vi "Measurement UI.vi"() -> ()   [LabVIEW 2024, in "Frequency Response (Discrete Sweep) UI.lvlib"]
uses:
  Frequency Response (Discrete Sweep) UI.lvlib
  <vilib>/gRPC/Generated APIs/ni/protobuf/types/RPC Messages/ni_protobuf_types_DoubleXYData.ctl
  <vilib>/gRPC/Generated APIs/ni/protobuf/types/ni.protobuf.types.lvlib
panel:
  out "RMS levels":cluster{"X":dbl[], "Y":dbl[]}[](graph)
  out "response RMS level":T1
  out "reference RMS level":T1
  out "Magnitude":cluster{"frequency":dbl[], "magnitude":dbl[]}(graph)
  out "FRF magnitude":T1
  out "Phase":cluster{"frequency":dbl[], "magnitude":dbl[]}(graph)
  out "FRF phase":T1
  out "Harmonic Distortion":cluster{"X":dbl[], "Y":dbl[]}[](graph)
  out "THDN":T1
  out "h5":T1
  out "h4":T1
  out "h3":T1
  out "h2":T1
  out "THD":T1
  out "waveforms file path":path
  in  "ai response":T2={"ai response channel (I/O)"="", "range"=3.16, "terminal configuration"=-1} {"terminal configuration" items=["Default"=-1, "RSE"=10083, "NRSE"=10078, "Differential"=10106, "Pseudodifferential"=12529]; "range" format="± %#_6f V"}
  in  "ai reference":T3={"ai reference channel (I/O)"="", "range"=3.16, "terminal configuration"=-1} {"terminal configuration" items=["Default"=-1, "RSE"=10083, "NRSE"=10078, "Differential"=10106, "Pseudodifferential"=12529]; "range" format="± %#_6f V"}
  in  "ao stimulus":T4={"ao stimulus channel (I/O)"="", "range"=3.16, "terminal configuration"=-1} {"terminal configuration" items=["Default"=-1, "RSE"=10083, "Differential"=10106, "Pseudodifferential"=12529]; "range" format="± %#_4f V"}
  in  "ai response terminal configuration":i32(ring)=-1 items=["Default"=-1, "RSE"=10083, "NRSE"=10078, "Differential"=10106, "Pseudodifferential"=12529]
  in  "ai response range":dbl=3.16 format="± %#_6f V"
  in  "ai response channel":string="Dev1/ai1"
  in  "ai reference terminal configuration":i32(ring)=-1 items=["Default"=-1, "RSE"=10083, "NRSE"=10078, "Differential"=10106, "Pseudodifferential"=12529]
  in  "ai ref range":dbl=3.16 format="± %#_6f V"
  in  "ai reference channel":string="Dev1/ai0"
  in  "ao terminal configuration":i32(ring)=-1 items=["Default"=-1, "RSE"=10083, "Differential"=10106, "Pseudodifferential"=12529]
  in  "ao range":dbl=3.16 format="± %#_4f V"
  in  "ao stimulus channel":string="Dev1/ao0"
  in  "sample rate":dbl=51200.0 format="%#_4p Hz"
  in  "amplitude":dbl=1.4142 format="%#_6f V"
  in  "profile":enum32{"Linear", "Logarithmic"}(ring)=enum."Logarithmic"
  in  "number of steps":i32=100 min=1
  in  "stop frequency":dbl=16000.0 format="%.2f Hz"
  in  "start frequency":dbl=31.25 format="%.2f Hz"
  in  "measurement cycles":i32=20 caption="cycles" min=1
  in  "measurement time":dbl=0.01 caption="time" format="%#_4f s"
  out "current frequency":dbl format="%#_g Hz"
  # "DAQ"
  # "Source"
  # "Measurement"
  # "Status"
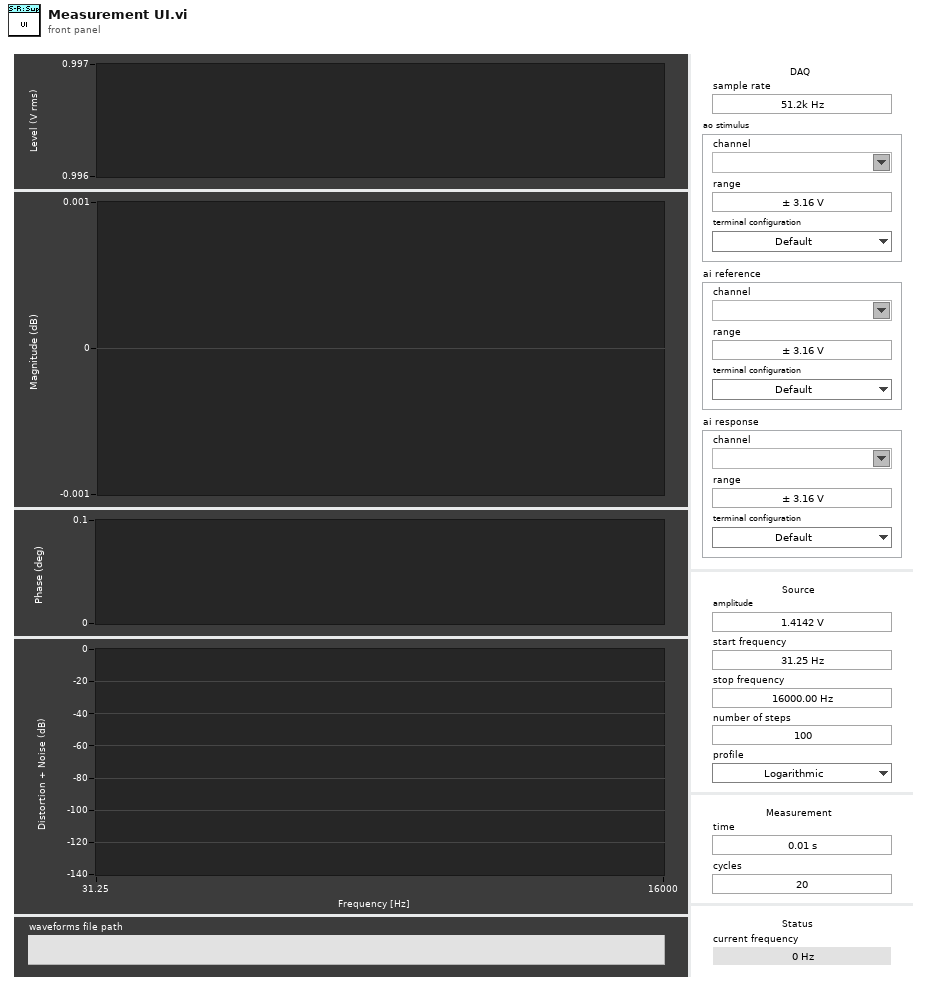
[diagram p1: front panel]
types:
  T1 = typedef "ni.protobuf.types.lvlib/ni_protobuf_types_DoubleXYData.ctl" = cluster{"x_data":dbl[], "y_data":dbl[]}
  T2 = cluster{"ai response channel (I/O)":tag, "range":dbl, "terminal configuration":i32}
  T3 = cluster{"ai reference channel (I/O)":tag, "range":dbl, "terminal configuration":i32}
  T4 = cluster{"ao stimulus channel (I/O)":tag, "range":dbl, "terminal configuration":i32}
  T5 = enum8{"Enabled", "Disabled", "Disabled and Grayed Out"}
  T6 = cluster{"I/O channel":tag, "range":dbl, "terminal configuration":i32}
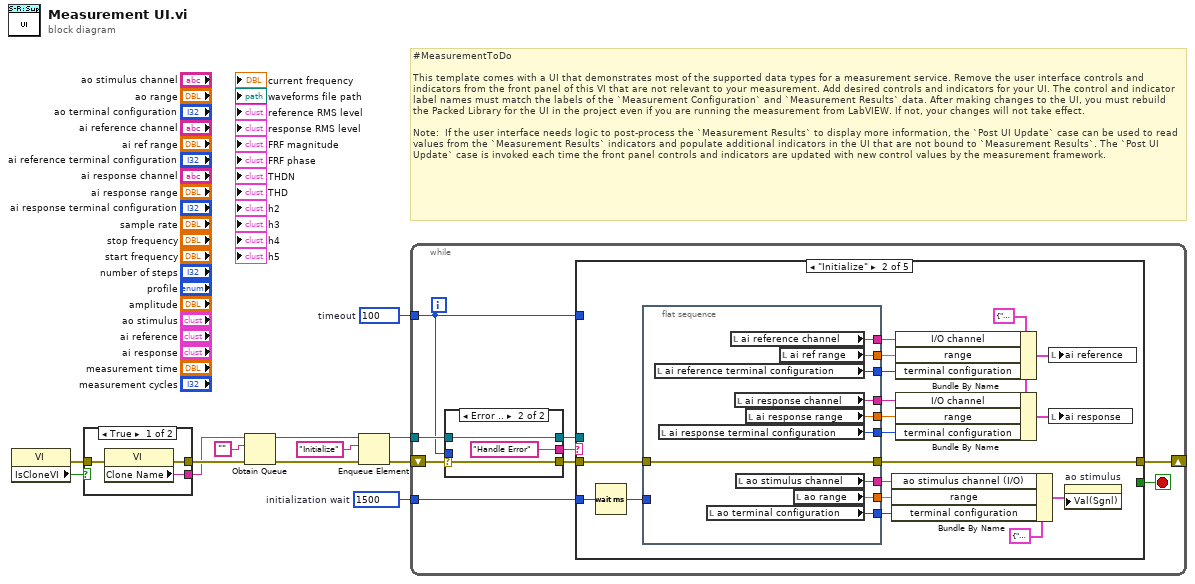
[diagram p0: block diagram]
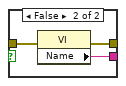
[diagram p2: hidden frame]
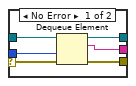
[diagram p3: hidden frame]
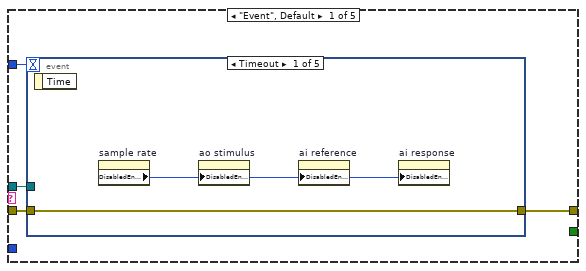
[diagram p4: hidden frame]
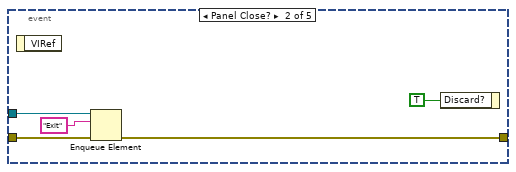
[diagram p5: hidden frame]
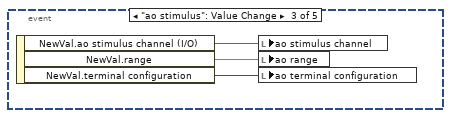
[diagram p6: hidden frame]
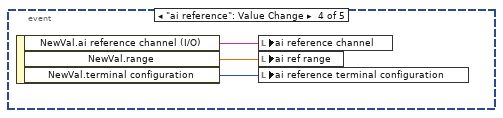
[diagram p7: hidden frame]
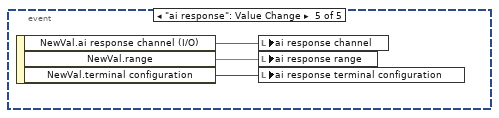
[diagram p8: hidden frame]
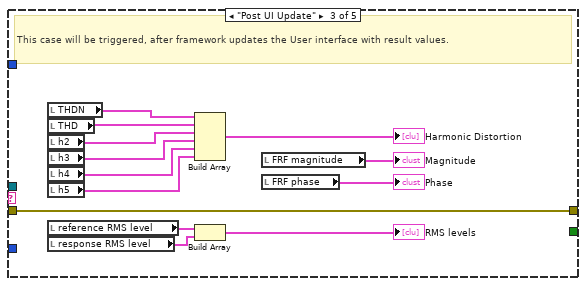
[diagram p9: hidden frame]
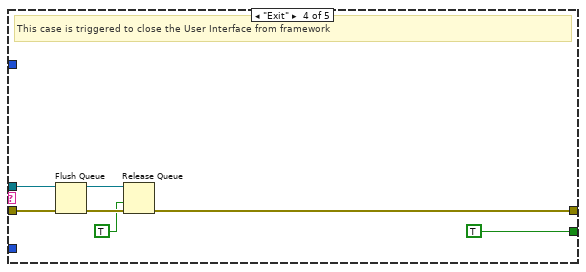
[diagram p10: hidden frame]
diagram:
  w1 = u32 1500  # initialization wait
  w2 = 100  # timeout
  # "#MeasurementToDo  \n\nThis template comes with a UI that demonstrates most of the supported data types for a measurement service. Remove the user interface controls and indicators from the front panel of this VI that are not relevant to your measurement. Add desired controls and indicators for your UI. The control and indicator label names must match the labels of the `Measurement Configuration` and `Measurement Results` data. After making changes to the UI, you must rebuild the Packed Library for the UI in the project even if you are running the measurement from LabVIEW. If not, your changes will not take effect.\n\nNote:  If the user interface needs logic to post-process the `Measurement Results` to display more information, the `Post UI Update` case can be used to read values from the `Measurement Results` indicators and populate additional indicators in the UI that are not bound to `Measurement Results`. The `Post UI Update` case is invoked each time the front panel controls and indicators are updated with new control values by the measurement framework."
  n1 = property class="VI"() -> (error out=w3:errorcluster, "IsCloneVI"=w4:bool)  [unwired: 2 in, 1 out]
  n2 = case shown="True" w4 {
    tunnel: [w15 w18] -> w12
    tunnel: [w14 w17] -> w11
    tunnel: w3 -> [w13 w16]
    frame True {
      n3 = property class="VI"(error in=w13) -> (error out=w15:errorcluster, "Clone Name"=w14:string)  [unwired: 1 in, 1 out]
    }
    frame False {
      n4 = property class="VI"(error in=w16) -> (error out=w18:errorcluster, "Name"=w17:string)  [unwired: 1 in, 1 out]
    }
  }
  n5 = Obtain Queue(name (unnamed)=w11, element data type="", error in (no error)=w12) -> (queue out=w8:refnum<queue>, error out=w10:errorcluster)  [unwired: 2 in, 1 out]
  n6 = Enqueue Element(queue=w8, element="Initialize", error in (no error)=w10) -> (queue out=w7:refnum<queue>, error out=w9:errorcluster)  [unwired: 1 in, 1 out]
  n7 = while {
    shift-right: [w22] -> _
    shift-left: w9 -> [w27]
    tunnel: w7 -> [w25]
    tunnel: w2 -> [w20]
    tunnel: w1 -> [w19]
    stop <- w21 stop-if-true
    n8 = case shown="Error .." w27 {
      selector: w27 -> [w33 w36]
      tunnel: [w32 w36] -> w26
      tunnel: w25 -> [w31 w35]
      tunnel: [w30 w35] -> w24
      tunnel: [w29 "Handle Error"] -> w23
      tunnel: w20 -> [w28 _]
      frame No Error {
        n9 = Dequeue Element(queue=w31, timeout in ms (-1)=w28, error in (no error)=w33) -> (queue out=w30:refnum<queue>, element=w29:string, error out=w32:errorcluster)  [unwired: 1 out]
      }
      frame Error {
      }
    }
    n10 = case shown="\"Initialize\"" w23 {
      tunnel: w26 -> [w39 w59 w97 w104 w105]
      tunnel: w24 -> [w38 _ _ w102 _]
      tunnel: [w40 w60 w97 w99 w105] -> w22
      tunnel: [_ _ _ TRUE _] -> w21
      tunnel: w20 -> [w37 _ _ _ _]
      tunnel: w19 -> [_ w58 _ _ _]
      frame "Event", Default {
        n11 = event shown="[0] Timeout" {
          selector: _ -> [_ _ _ _ _]
          dyn-events: _ -> [_ _ _ _ _]
          timeout: w37 -> [_ _ _ _ _]
          tunnel: [w42 w45 _ _ _] -> w40
          tunnel: w39 -> [w42 w46 _ _ _]
          tunnel: w38 -> [_ w44 _ _ _]
          event Timeout {
            n12 = event-data() -> ()  [unwired: 1 in, 1 out]
            n13 = property on="sample rate" class="DigNum (strict)"() -> ("DisabledEnum"=w41:T5)  [unwired: 2 in, 2 out]
            n14 = property on="ao stimulus" class="Clust (strict)"("DisabledEnum"=w41) -> ()  [unwired: 2 in, 2 out]
            n15 = property on="ai reference" class="Clust (strict)"("DisabledEnum"=w41) -> ()  [unwired: 2 in, 2 out]
            n16 = property on="ai response" class="Clust (strict)"("DisabledEnum"=w41) -> ()  [unwired: 2 in, 2 out]
          }
          event Panel Close? {
            n17 = event-data() -> ()  [unwired: 1 in, 1 out]
            n18 = Enqueue Element(queue=w44, element="Exit", error in (no error)=w46) -> (error out=w45:errorcluster)  [unwired: 1 in, 2 out]
            n19 = event-data("Discard?"=TRUE) -> ()  [unwired: 1 in, 1 out]
          }
          event "ao stimulus": Value Change {
            n20 = event-data() -> ("NewVal.ao stimulus channel (I/O)"=w50:tag, "NewVal.range"=w49:dbl, "NewVal.terminal configuration"=w48:i32)  [unwired: 1 in]
            n21 = local write "ao stimulus channel"(w50) -> ()
            n22 = local write "ao range"(w49) -> ()
            n23 = local write "ao terminal configuration"(w48) -> ()
          }
          event "ai reference": Value Change {
            n24 = event-data() -> ("NewVal.ai reference channel (I/O)"=w53:tag, "NewVal.range"=w52:dbl, "NewVal.terminal configuration"=w51:i32)  [unwired: 1 in]
            n25 = local write "ai reference channel"(w53) -> ()
            n26 = local write "ai ref range"(w52) -> ()
            n27 = local write "ai reference terminal configuration"(w51) -> ()
          }
          event "ai response": Value Change {
            n28 = event-data() -> ("NewVal.ai response channel (I/O)"=w56:tag, "NewVal.range"=w55:dbl, "NewVal.terminal configuration"=w54:i32)  [unwired: 1 in]
            n29 = local write "ai response channel"(w56) -> ()
            n30 = local write "ai response range"(w55) -> ()
            n31 = local write "ai response terminal configuration"(w54) -> ()
          }
        }
      }
      frame "Initialize" {
        w61 = T6 {"I/O channel"="", "range"=31.25, "terminal configuration"=-1} ("ai reference")
        n32 = Wait (ms)(milliseconds to wait=w58) -> (millisecond timer value=w57:u32)
        n33 = flat-sequence {
          tunnel: [w84] -> w73
          tunnel: [w83] -> w72
          tunnel: [w82] -> w71
          tunnel: [w81] -> w69
          tunnel: [w80] -> w67
          tunnel: [w79] -> w66
          tunnel: [w78] -> w65
          tunnel: [w77] -> w64
          tunnel: [w76] -> w62
          tunnel: [w75] -> w60
          tunnel: w59 -> [w75]
          tunnel: w57 -> [_]
          frame #0 {
            n34 = local read "ai reference terminal configuration"() -> (w79:i32)
            n35 = local read "ai response terminal configuration"() -> (w78:i32)
            n36 = local read "ao terminal configuration"() -> (w82:i32)
            n37 = local read "ai reference channel"() -> (w80:string)
            n38 = local read "ai response channel"() -> (w77:string)
            n39 = local read "ao stimulus channel"() -> (w84:string)
            n40 = local read "ai response range"() -> (w76:dbl)
            n41 = local read "ai ref range"() -> (w81:dbl)
            n42 = local read "ao range"() -> (w83:dbl)
          }
        }
        n43 = Bundle By Name(cluster=T4 {"ao stimulus channel (I/O)"="", "range"=0.0, "terminal configuration"=0} ("Value (Signaling)"), "ao stimulus channel (I/O)"=w73, "range"=w72, "terminal configuration"=w71) -> (w70:T4)
        n44 = Bundle By Name(cluster=w61, "I/O channel"=w67, "range"=w69, "terminal configuration"=w66) -> (w68:T6)
        n45 = Bundle By Name(cluster=w61, "I/O channel"=w64, "range"=w62, "terminal configuration"=w65) -> (w63:T6)
        n46 = local write "ai reference"(w68) -> ()
        n47 = local write "ai response"(w63) -> ()
        n48 = property on="ao stimulus" class="Clust (strict)"("Val(Sgnl)"=w70) -> ()  [unwired: 2 in, 2 out]
      }
      frame "Post UI Update" {
        # "This case will be triggered, after framework updates the User interface with result values."
        n49 = local read "THDN"() -> (w91:T1)
        n50 = local read "THD"() -> (w90:T1)
        n51 = local read "h2"() -> (w89:T1)
        n52 = local read "h3"() -> (w88:T1)
        n53 = local read "h4"() -> (w87:T1)
        n54 = local read "h5"() -> (w86:T1)
        n55 = local read "reference RMS level"() -> (w96:T1)
        n56 = local read "response RMS level"() -> (w95:T1)
        n57 = Build Array(w91, w90, w89, w88, w87, w86) -> (→"Harmonic Distortion":T1[])
        n58 = Build Array(w96, w95) -> (→"RMS levels":T1[])
        n59 = local read "FRF magnitude"() -> (→"Magnitude":T1)
        n60 = local read "FRF phase"() -> (→"Phase":T1)
      }
      frame "Exit" {
        # "This case is triggered to close the User Interface from framework"
        n61 = Flush Queue(queue=w102, error in (no error)=w104) -> (queue out=w101:refnum<queue>, error out=w100:errorcluster)  [unwired: 1 out]
        n62 = Release Queue(queue=w101, force destroy? (F)=TRUE, error in (no error)=w100) -> (error out=w99:errorcluster)  [unwired: 2 out]
      }
      frame "Handle Error" {
      }
    }
  }
